vi "Test Serialize Variant Attributes.vi"(8 "error in (no error)":errorcluster) -> (0 "error out":errorcluster)   [LabVIEW 2015]
uses:
  src/Serializer/JSON Serializer/JSON Serializer.lvclass
  <vilib>/addons/_JKI Toolkits/Caraya/classes/Test/Test.lvclass
  <vilib>/addons/_JKI Toolkits/Caraya/classes/Assert/Assert.lvclass
panel:
  out "String":string
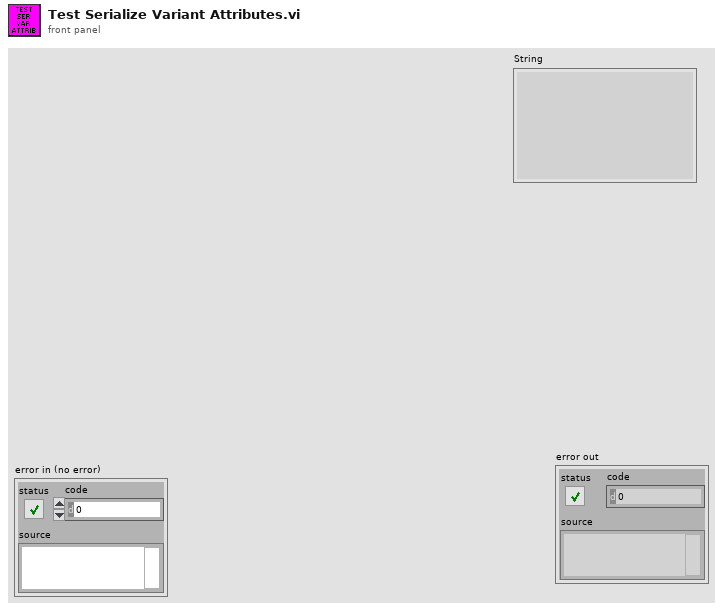
[diagram p1: front panel]
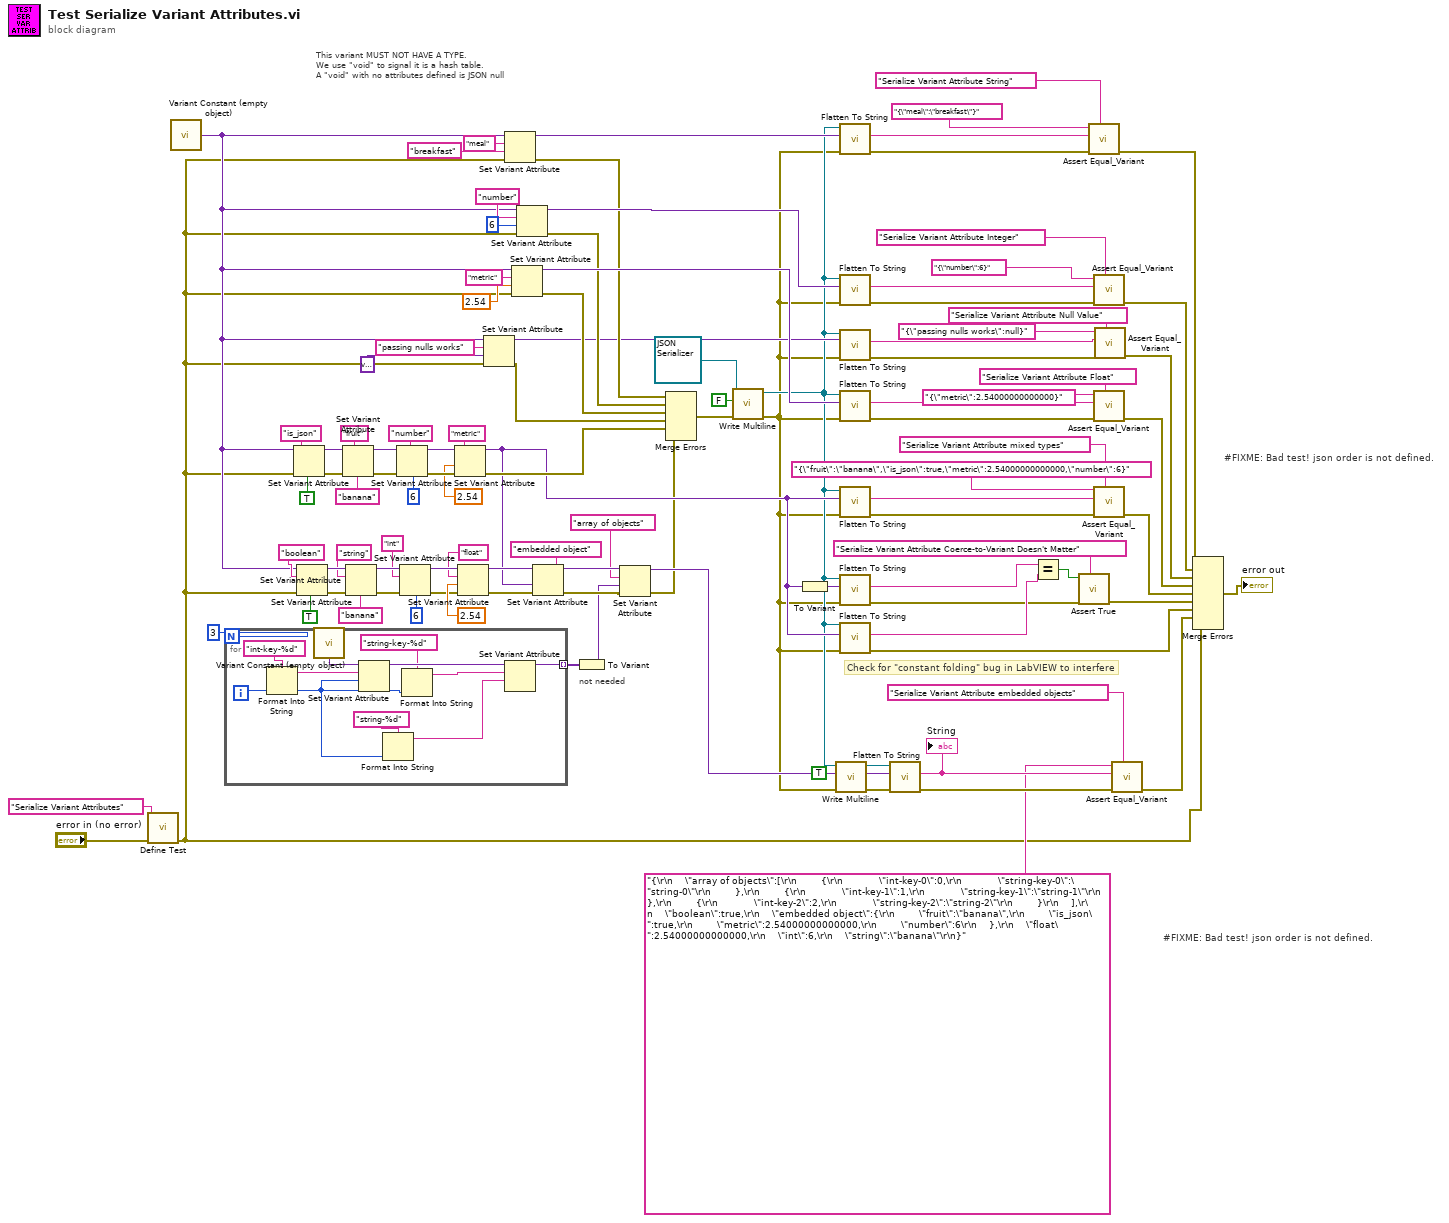
[diagram p0: block diagram]
diagram:
  # "#FIXME: Bad test! json order is not defined."
  # "not needed"
  # "#FIXME: Bad test! json order is not defined."
  # "This variant MUST NOT HAVE A TYPE.\nWe use \"void\" to signal it is a hash table.\nA \"void\" with no attributes defined is JSON null"
  # "Check for \"constant folding\" bug in LabVIEW to interfere"
  n1 = call <vilib>:"Define Test.vi"("error in (no error)"="error in (no error)", "Label (VI Title)"="Serialize Variant Attributes") -> ("error out"=w1:errorcluster)  [unwired: 9 in]
  n2 = call "Variant Constant (empty object).vi"() -> ("Empty Object"=w24:variant)  [unwired: 2 in]
  n3 = for {
    N: 3 -> [_]
    tunnel: [w115] -> w10 mode=indexing
    i -> [w111]
    n4 = Format Into String(format string="int-key-%d", w111) -> (resulting string=w113:string)  [unwired: 2 in, 1 out]
    n5 = call "Variant Constant (empty object).vi"() -> ("Empty Object"=w117:variant)  [unwired: 2 in]
    n6 = Set Variant Attribute(Variant=w117, name=w113, value=w111) -> (Variant out=w116:variant)  [unwired: 1 in, 2 out]
    n7 = Format Into String(format string="string-%d", w111) -> (resulting string=w109:string)  [unwired: 2 in, 1 out]
    n8 = Format Into String(format string="string-key-%d", w111) -> (resulting string=w112:string)  [unwired: 2 in, 1 out]
    n9 = Set Variant Attribute(Variant=w116, name=w112, value=w109) -> (Variant out=w115:variant)  [unwired: 1 in, 2 out]
  }
  n10 = Set Variant Attribute(Variant=w24, name="is_json", value=TRUE, error in=w1) -> (Variant out=w77:variant, error out=w108:errorcluster)  [unwired: 1 out]
  n11 = Set Variant Attribute(Variant=w24, name="boolean", value=TRUE, error in=w1) -> (Variant out=w35:variant, error out=w25:errorcluster)  [unwired: 1 out]
  n12 = Set Variant Attribute(Variant=w77, name="fruit", value="banana" ("name"), error in=w108) -> (Variant out=w76:variant, error out=w107:errorcluster)  [unwired: 1 out]
  n13 = Set Variant Attribute(Variant=w35, name="string", value="banana" ("name"), error in=w25) -> (Variant out=w36:variant, error out=w26:errorcluster)  [unwired: 1 out]
  n14 = Set Variant Attribute(Variant=w76, name="number", value=6, error in=w107) -> (Variant out=w75:variant, error out=w106:errorcluster)  [unwired: 1 out]
  n15 = Set Variant Attribute(Variant=w36, name="int", value=6, error in=w26) -> (Variant out=w37:variant, error out=w27:errorcluster)  [unwired: 1 out]
  n16 = Set Variant Attribute(Variant=w75, name="metric", value=2.54, error in=w106) -> (Variant out=w20:variant, error out=w49:errorcluster)  [unwired: 1 out]
  n17 = Set Variant Attribute(Variant=w37, name="float", value=2.54, error in=w27) -> (Variant out=w22:variant, error out=w23:errorcluster)  [unwired: 1 out]
  n18 = Set Variant Attribute(Variant=w24, name="passing nulls works", value=variant, error in=w1) -> (Variant out=w43:variant, error out=w46:errorcluster)  [unwired: 1 out]
  n19 = Set Variant Attribute(Variant=w24, name="meal", value="breakfast" ("name"), error in=w1) -> (Variant out=w74:variant, error out=w62:errorcluster)  [unwired: 1 out]
  n20 = Set Variant Attribute(Variant=w24, name="metric", value=2.54, error in=w1) -> (Variant out=w69:variant, error out=w60:errorcluster)  [unwired: 1 out]
  n21 = Set Variant Attribute(Variant=w24, name="number", value=6, error in=w1) -> (Variant out=w73:variant, error out=w61:errorcluster)  [unwired: 1 out]
  n22 = Set Variant Attribute(Variant=w22, name="embedded object", value=w20, error in=w23) -> (Variant out=w18:variant, error out=w19:errorcluster)  [unwired: 1 out]
  n23 = To Variant(anything=w10) -> (Variant=w11:variant)
  n24 = Set Variant Attribute(Variant=w18, name="array of objects", value=w11, error in=w19) -> (Variant out=w13:variant, error out=w9:errorcluster)  [unwired: 1 out]
  n25 = Merge Errors(w62, w61, w60, w46, w49, w9) -> (w57:errorcluster)
  n26 = call-dynamic "Write Multiline.vi"("error in (no error)"=w57, "Multiline"=FALSE, "JSON Serializer in"=refnum<class "JSON Serializer.lvclass"> refnum ("JKI JSON Serialization.lvlib:JSON Serializer.lvclass")) -> ("error out"=w6:errorcluster, "JSON Serializer out"=w8:refnum<class "JSON Serializer.lvclass">)  [unwired: 7 in]
  n27 = To Variant(anything=w20) -> (Variant=w72:variant)
  n28 = call-dynamic "Write Multiline.vi"("error in (no error)"=w6, "Multiline"=TRUE, "JSON Serializer in"=w8) -> ("error out"=w5:errorcluster, "JSON Serializer out"=w7:refnum<class "JSON Serializer.lvclass">)  [unwired: 7 in]
  n29 = call-dynamic "Flatten To String.vi"("error in (no error)"=w6, "Variant"=w74, "JSON Serializer in"=w8) -> ("error out"=w99:errorcluster, "String"=w97:string)  [unwired: 6 in, 1 out]
  n30 = call-dynamic "Flatten To String.vi"("error in (no error)"=w6, "Variant"=w73, "JSON Serializer in"=w8) -> ("error out"=w93:errorcluster, "String"=w92:string)  [unwired: 6 in, 1 out]
  n31 = call-dynamic "Flatten To String.vi"("error in (no error)"=w6, "Variant"=w43, "JSON Serializer in"=w8) -> ("error out"=w42:errorcluster, "String"=w40:string)  [unwired: 6 in, 1 out]
  n32 = call-dynamic "Flatten To String.vi"("error in (no error)"=w6, "Variant"=w69, "JSON Serializer in"=w8) -> ("error out"=w94:errorcluster, "String"=w52:string)  [unwired: 6 in, 1 out]
  n33 = call-dynamic "Flatten To String.vi"("error in (no error)"=w6, "Variant"=w20, "JSON Serializer in"=w8) -> ("error out"=w59:errorcluster, "String"=w56:string)  [unwired: 6 in, 1 out]
  n34 = call-dynamic "Flatten To String.vi"("error in (no error)"=w6, "Variant"=w72, "JSON Serializer in"=w8) -> ("error out"=w65:errorcluster, "String"=w68:string)  [unwired: 6 in, 1 out]
  n35 = call-dynamic "Flatten To String.vi"("error in (no error)"=w6, "Variant"=w20, "JSON Serializer in"=w8) -> ("error out"=w55:errorcluster, "String"=w67:string)  [unwired: 6 in, 1 out]
  n36 = call-dynamic "Flatten To String.vi"("error in (no error)"=w5, "Variant"=w13, "JSON Serializer in"=w7) -> ("error out"=w14:errorcluster, "String"=w3:string)  [unwired: 6 in, 1 out]
  "String" <- w3
  n37 = Equal?(x=w68, y=w67) -> (x = y?=w66:bool)
  n38 = call <vilib>:"Assert True.vi"("Label"="Serialize Variant Attribute Coerce-to-Variant Doesn't Matter", "error in (no error)"=w65, "True?"=w66) -> ("error out"=w54:errorcluster)  [unwired: 8 in]
  n39 = call <vilib>:"Assert Equal_Variant.vi"("Label"="Serialize Variant Attribute String", "error in (no error)"=w99, "Y"=w97, "X"="{\"meal\":\"breakfast\"}" ("String 2")) -> ("error out"=w96:errorcluster)  [unwired: 7 in]
  n40 = call <vilib>:"Assert Equal_Variant.vi"("Label"="Serialize Variant Attribute Integer", "error in (no error)"=w93, "Y"=w92, "X"="{\"number\":6}" ("String")) -> ("error out"=w45:errorcluster)  [unwired: 7 in]
  n41 = call <vilib>:"Assert Equal_Variant.vi"("Label"="Serialize Variant Attribute Float", "error in (no error)"=w94, "Y"=w52, "X"="{\"metric\":2.54000000000000}" ("String 2")) -> ("error out"=w100:errorcluster)  [unwired: 7 in]
  n42 = call <vilib>:"Assert Equal_Variant.vi"("Label"="Serialize Variant Attribute mixed types", "error in (no error)"=w59, "Y"=w56, "X"="{\"fruit\":\"banana\",\"is_json\":true,\"metric\":2.54000000000000,\"number\":6}" ("String")) -> ("error out"=w53:errorcluster)  [unwired: 7 in]
  n43 = call <vilib>:"Assert Equal_Variant.vi"("Label"="Serialize Variant Attribute Null Value", "error in (no error)"=w42, "Y"=w40, "X"="{\"passing nulls works\":null}" ("String")) -> ("error out"=w44:errorcluster)  [unwired: 7 in]
  n44 = call <vilib>:"Assert Equal_Variant.vi"("Label"="Serialize Variant Attribute embedded objects", "error in (no error)"=w14, "Y"=w3, "X"="{\r\n    \"array of objects\":[\r\n        {\r\n            \"int-key-0\":0,\r\n            \"string-key-0\":\"string-0\"\r\n        },\r\n        {\r\n            \"int-key-1\":1,\r\n            \"string-key-1\":\"string-1\"\r\n        },\r\n        {\r\n            \"int-key-2\":2,\r\n            \"string-key-2\":\"string-2\"\r\n        }\r\n    ],\r\n    \"boolean\":true,\r\n    \"embedded object\":{\r\n        \"fruit\":\"banana\",\r\n        \"is_json\":true,\r\n        \"metric\":2.54000000000000,\r\n        \"number\":6\r\n    },\r\n    \"float\":2.54000000000000,\r\n    \"int\":6,\r\n    \"string\":\"banana\"\r\n}" ("String")) -> ("error out"=w12:errorcluster)  [unwired: 7 in]
  n45 = Merge Errors(w96, w45, w44, w100, w53, w54, w55, w12, w1) -> (→"error out":errorcluster)
